vi "UDP Heartbeat Globals.vi"() -> ()   [LabVIEW 2013]
panel:
  out "State":bool
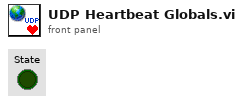
[diagram p1: front panel]
diagram:
